vi "FindMultiVar.vi"(6 "Write?":bool, 7 "Abs_Type":refnum<class "Abs_Type.lvclass">, 8 "error in (no error)":errorcluster, 9 "Tag":string[](array[string]), 10 "Abs_Type Default":refnum<class "Abs_Type.lvclass">[](array[class]), 11 "Var Bus in":refnum<class "Omni_Bus.lvclass">) -> (0 "error out":errorcluster, 1 "Updated Tags":bool[](array[boolean]), 2 "Abs_Type Found":refnum<class "Abs_Type.lvclass">[](array[class]), 3 "Var Bus out":refnum<class "Omni_Bus.lvclass">)   [LabVIEW 2021, in "Omni_Bus.lvclass"]
uses:
  Omni_Bus.lvclass
  <vilib>/TSA/Abstract Data Classes/Abs_Types/Type/Abs_Type.lvclass/Abs_Type.ctl
  Omni_Bus.lvclass/Omni_Bus.ctl
  <vilib>/Utility/error.llb/Clear Errors.vi
  Properties/Read Var Map.vi
  <vilib>/TSA/Abstract Data Classes/Abs_Types/Type/Properties/Read Tag.vi
  <vilib>/TSA/Abstract Data Classes/Abs_Types/Value/Abs_Value.lvclass
  C:/Program Files (x86)/National Instruments/LabVIEW 2021/vi.lib/TSA/Abstract Data Classes/Abs_Types/Type/Abs_Type.lvclass
  Check For Read Only Error.vi
  Incorrect Tag String Error.vi
  <vilib>/TSA/Abstract Data Classes/Abs_Types/Type/Abs_Type.lvclass
panel:
  # "can only be \ntrue if a value type"
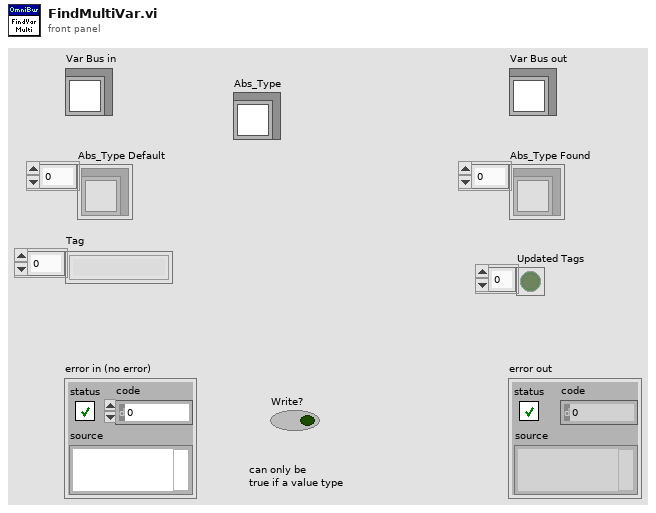
[diagram p1: front panel]
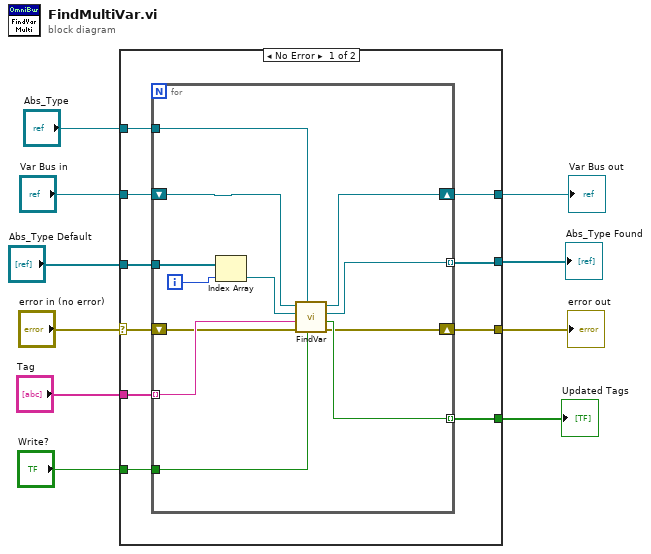
[diagram p0: block diagram]
diagram:
  n1 = case shown="No Error" "error in (no error)" {
    selector: "error in (no error)" -> [w20 w35]
    tunnel: [w17 w35] -> w9
    tunnel: [w16 w34] -> w7
    tunnel: "Var Bus in" -> [w19 w34]
    tunnel: "Tag" -> [w14 _]
    tunnel: [w18 w33] -> w5
    tunnel: "Abs_Type Default" -> [w15 w33]
    tunnel: "Write?" -> [w13 _]
    tunnel: [w12 _] -> w2
    tunnel: "Abs_Type" -> [w11 _]
    frame No Error {
      n2 = for {
        tunnel: w14 -> [w32] mode=indexing
        tunnel: w13 -> [w31]
        shift-right: [w24] -> w17
        shift-left: w20 -> [w25]
        shift-right: [w26] -> w16
        shift-left: w19 -> [w27]
        tunnel: [w30] -> w12 mode=indexing
        tunnel: w15 -> [w29]
        tunnel: [w22] -> w18 mode=indexing
        tunnel: w11 -> [w21]
        i -> [w28]
        n3 = Index Array(array=w29, index=w28) -> (element=w23:refnum<class "Abs_Type.lvclass">)
        n4 = call "FindVar.vi"("Write?"=w31, "Abs_Type"=w21, "error in (no error)"=w25, "Tag"=w32, "Abs_Type Default"=w23, "Var Bus in"=w27) -> ("error out"=w24:errorcluster, "Updated Tag"=w30:bool, "Abs_Type Found"=w22:refnum<class "Abs_Type.lvclass">, "Var Bus out"=w26:refnum<class "Omni_Bus.lvclass">)  [unwired: 2 in]
      }
    }
    frame Error {
    }
  }
  "error out" <- w9
  "Var Bus out" <- w7
  "Abs_Type Found" <- w5
  "Updated Tags" <- w2
